vi "VMC-1.vi"(11 "数组":u8[](array[numeric])) -> (1 "传感器信号":cluster{"陀螺温度":i16, "加速度计温度":i16}, 2 "加速度":cluster{"X轴加速度":i32, "Y轴加速度":i32, "Z轴加速度":i32}, 3 "角速度":cluster{"X轴角速度":i32, "Y轴角速度":i32, "Z轴角速度":i32}, 4 "时间增量":i8, 5 "视速度增量":cluster{"X轴增量":i16, "Y轴增量":i16, "Z轴增量":i16}, 6 "角度增量":cluster{"X轴角增量":i16, "Y轴角增量":i16, "Z轴角增量":i16})   [LabVIEW 2012]
uses:
  index-i16.vi
  index-i32.vi
  index-i8.vi
  XX-I32.vi
  XX-I16.vi
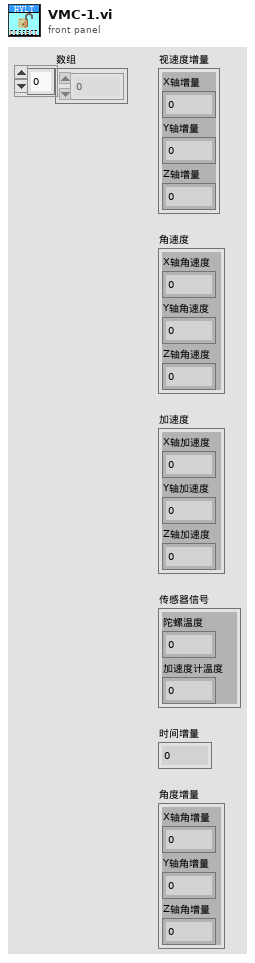
[diagram p1: front panel]
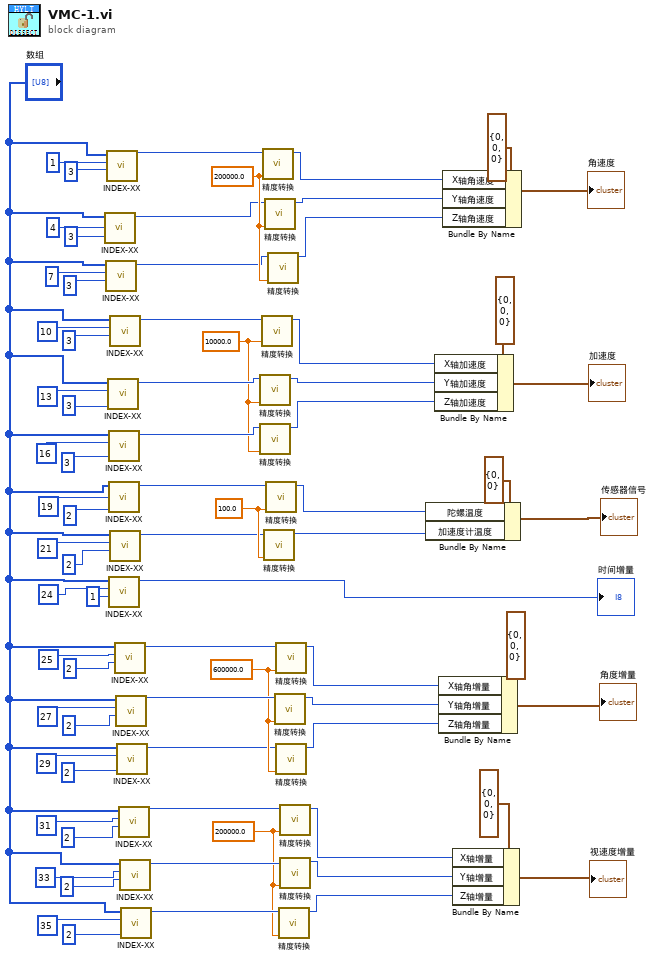
[diagram p0: block diagram]
diagram:
  w1 = 200000.0 ("单位")
  w10 = 600000.0 ("单位")
  w17 = 100.0 ("单位")
  w20 = 10000.0 ("单位")
  w31 = 200000.0 ("单位")
  n1 = call-poly "INDEX-XX.vi"("长度"=3, "索引"=4, "数组"="数组") -> ("数值输出"=w30:i32)  [unwired: 8 in]
  n2 = call-poly "INDEX-XX.vi"("长度"=3, "索引"=7, "数组"="数组") -> ("数值输出"=w29:i32)  [unwired: 8 in]
  n3 = call-poly "INDEX-XX.vi"("长度"=3, "索引"=1, "数组"="数组") -> ("数值输出"=w33:i32)  [unwired: 8 in]
  n4 = call-poly "INDEX-XX.vi"("长度"=3, "索引"=13, "数组"="数组") -> ("数值输出"=w22:i32)  [unwired: 8 in]
  n5 = call-poly "INDEX-XX.vi"("长度"=3, "索引"=16, "数组"="数组") -> ("数值输出"=w21:i32)  [unwired: 8 in]
  n6 = call-poly "INDEX-XX.vi"("长度"=2, "索引"=19, "数组"="数组") -> ("数值输出"=w19:i16)  [unwired: 8 in]
  n7 = call-poly "INDEX-XX.vi"("长度"=1, "索引"=24, "数组"="数组") -> ("数值输出"=→"时间增量":i8)  [unwired: 8 in]
  n8 = call-poly "INDEX-XX.vi"("长度"=3, "索引"=10, "数组"="数组") -> ("数值输出"=w26:i32)  [unwired: 8 in]
  n9 = call-poly "INDEX-XX.vi"("长度"=2, "索引"=21, "数组"="数组") -> ("数值输出"=w16:i16)  [unwired: 8 in]
  n10 = call-poly "INDEX-XX.vi"("长度"=2, "索引"=25, "数组"="数组") -> ("数值输出"=w14:i16)  [unwired: 8 in]
  n11 = call-poly "INDEX-XX.vi"("长度"=2, "索引"=27, "数组"="数组") -> ("数值输出"=w12:i16)  [unwired: 8 in]
  n12 = call-poly "INDEX-XX.vi"("长度"=2, "索引"=29, "数组"="数组") -> ("数值输出"=w9:i16)  [unwired: 8 in]
  n13 = call-poly "INDEX-XX.vi"("长度"=2, "索引"=31, "数组"="数组") -> ("数值输出"=w7:i16)  [unwired: 8 in]
  n14 = call-poly "INDEX-XX.vi"("长度"=2, "索引"=33, "数组"="数组") -> ("数值输出"=w5:i16)  [unwired: 8 in]
  n15 = call-poly "INDEX-XX.vi"("长度"=2, "索引"=35, "数组"="数组") -> ("数值输出"=w3:i16)  [unwired: 8 in]
  n16 = call-poly "精度转换.vi"("单位"=w20, "数值输入"=w22) -> ("输出"=w24:i32)  [unwired: 9 in]
  n17 = call-poly "精度转换.vi"("单位"=w20, "数值输入"=w21) -> ("输出"=w23:i32)  [unwired: 9 in]
  n18 = call-poly "精度转换.vi"("单位"=w20, "数值输入"=w26) -> ("输出"=w25:i32)  [unwired: 9 in]
  n19 = call-poly "精度转换.vi"("单位"=w31, "数值输入"=w33) -> ("输出"=w32:i32)  [unwired: 9 in]
  n20 = call-poly "精度转换.vi"("单位"=w17, "数值输入"=w16) -> ("输出"=w15:i16)  [unwired: 9 in]
  n21 = call-poly "精度转换.vi"("单位"=w31, "数值输入"=w30) -> ("输出"=w28:i32)  [unwired: 9 in]
  n22 = call-poly "精度转换.vi"("单位"=w17, "数值输入"=w19) -> ("输出"=w18:i16)  [unwired: 9 in]
  n23 = call-poly "精度转换.vi"("单位"=w31, "数值输入"=w29) -> ("输出"=w27:i32)  [unwired: 9 in]
  n24 = call-poly "精度转换.vi"("单位"=w10, "数值输入"=w12) -> ("输出"=w11:i16)  [unwired: 9 in]
  n25 = call-poly "精度转换.vi"("单位"=w10, "数值输入"=w14) -> ("输出"=w13:i16)  [unwired: 9 in]
  n26 = call-poly "精度转换.vi"("单位"=w10, "数值输入"=w9) -> ("输出"=w8:i16)  [unwired: 9 in]
  n27 = call-poly "精度转换.vi"("单位"=w1, "数值输入"=w3) -> ("输出"=w2:i16)  [unwired: 9 in]
  n28 = call-poly "精度转换.vi"("单位"=w1, "数值输入"=w7) -> ("输出"=w6:i16)  [unwired: 9 in]
  n29 = call-poly "精度转换.vi"("单位"=w1, "数值输入"=w5) -> ("输出"=w4:i16)  [unwired: 9 in]
  n30 = Bundle By Name(cluster=cluster{"陀螺温度":i16, "加速度计温度":i16} {"陀螺温度"=0, "加速度计温度"=0} ("传感器信号"), "陀螺温度"=w18, "加速度计温度"=w15) -> (→"传感器信号":cluster{"陀螺温度":i16, "加速度计温度":i16})
  n31 = Bundle By Name(cluster=cluster{"X轴加速度":i32, "Y轴加速度":i32, "Z轴加速度":i32} {"X轴加速度"=0, "Y轴加速度"=0, "Z轴加速度"=0} ("加速度"), "X轴加速度"=w25, "Y轴加速度"=w24, "Z轴加速度"=w23) -> (→"加速度":cluster{"X轴加速度":i32, "Y轴加速度":i32, "Z轴加速度":i32})
  n32 = Bundle By Name(cluster=cluster{"X轴角增量":i16, "Y轴角增量":i16, "Z轴角增量":i16} {"X轴角增量"=0, "Y轴角增量"=0, "Z轴角增量"=0} ("角度增量"), "X轴角增量"=w13, "Y轴角增量"=w11, "Z轴角增量"=w8) -> (→"角度增量":cluster{"X轴角增量":i16, "Y轴角增量":i16, "Z轴角增量":i16})
  n33 = Bundle By Name(cluster=cluster{"X轴角速度":i32, "Y轴角速度":i32, "Z轴角速度":i32} {"X轴角速度"=0, "Y轴角速度"=0, "Z轴角速度"=0} ("角速度"), "X轴角速度"=w32, "Y轴角速度"=w28, "Z轴角速度"=w27) -> (→"角速度":cluster{"X轴角速度":i32, "Y轴角速度":i32, "Z轴角速度":i32})
  n34 = Bundle By Name(cluster=cluster{"X轴增量":i16, "Y轴增量":i16, "Z轴增量":i16} {"X轴增量"=0, "Y轴增量"=0, "Z轴增量"=0} ("视速度增量"), "X轴增量"=w6, "Y轴增量"=w4, "Z轴增量"=w2) -> (→"视速度增量":cluster{"X轴增量":i16, "Y轴增量":i16, "Z轴增量":i16})
